vi "Configure Session.vi"(8 "error in":errorcluster, 11 "Plugin in":refnum<class "Sequencer with Output Values.lvclass">) -> (0 "error out":errorcluster, 3 "Plugin out":refnum<class "Sequencer with Output Values.lvclass">)   [LabVIEW 2024, in "Sequencer with Output Values.lvlib" / "Sequencer with Output Values.lvclass"]
uses:
  Sequencer with Output Values.lvclass
  C:/Program Files/National Instruments/LabVIEW 2024/vi.lib/FlexLogger/SDK/PluginSDK.lvlibp/PEFClasses/SDK/Plugin/Plugin.lvclass
  Sequencer with Output Values.lvclass/Sequencer with Output Values.ctl
  Global Strings.vi
  <vilib>/FlexLogger/SDK/PluginSDK.lvlibp/PEFClasses/SDK/Plugin/ParameterAccess/Read I32.vi
  <vilib>/FlexLogger/SDK/PluginSDK.lvlibp/PEFClasses/SDK/Plugin/ParameterAccess/Write I32.vi
  <vilib>/FlexLogger/SDK/PluginSDK.lvlibp/PEFClasses/SDK/Plugin/ParameterAccess/Read DBL.vi
  <vilib>/FlexLogger/SDK/PluginSDK.lvlibp/PEFClasses/SDK/Plugin/ParameterAccess/Read Boolean.vi
  <vilib>/FlexLogger/SDK/PluginSDK.lvlibp/PEFClasses/SDK/Plugin/Plugin.lvclass
  C:/Program Files/National Instruments/LabVIEW 2024/vi.lib/FlexLogger/SDK/PluginSDK.lvlibp/PEFClasses/SDK/Processing Element/Processing Element.lvclass
  C:/dev/niflexlogger-plugins/plugins/Sequencer with Output Values/source/Sequencer with Output Values/Sequencer with Output Values.lvclass
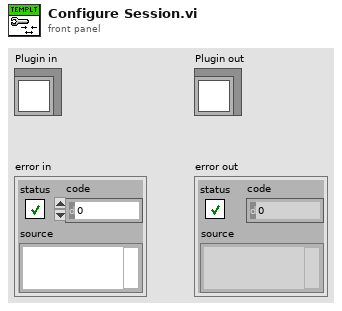
[diagram p1: front panel]
types:
  T1 = typedef "Sequencer with Output Values.lvlib/Sequencer with Output Values.lvclass/Params.ctl" = cluster{"Step Values":T2[], "Only Execute When Test Running":bool, "Current Sequence ID":u32, "Total Iterations":u32, "Last Timestamp":timestamp, "Number of Sequence Steps":i32, "Number of Analog Channels":i32, "Number of Digital Channels":i32, "Delay Before Starting Sequence":dbl}
  T2 = typedef "Step Settings.ctl" = cluster{"Duration":dbl, "Mode":string, "Delay Between Values":dbl, "Analog Values":string[], "Digital Values":string[]}
  T3 = cluster{"Number of Sequence Steps":i32, "Number of Analog Channels":i32, "Number of Digital Channels":i32}
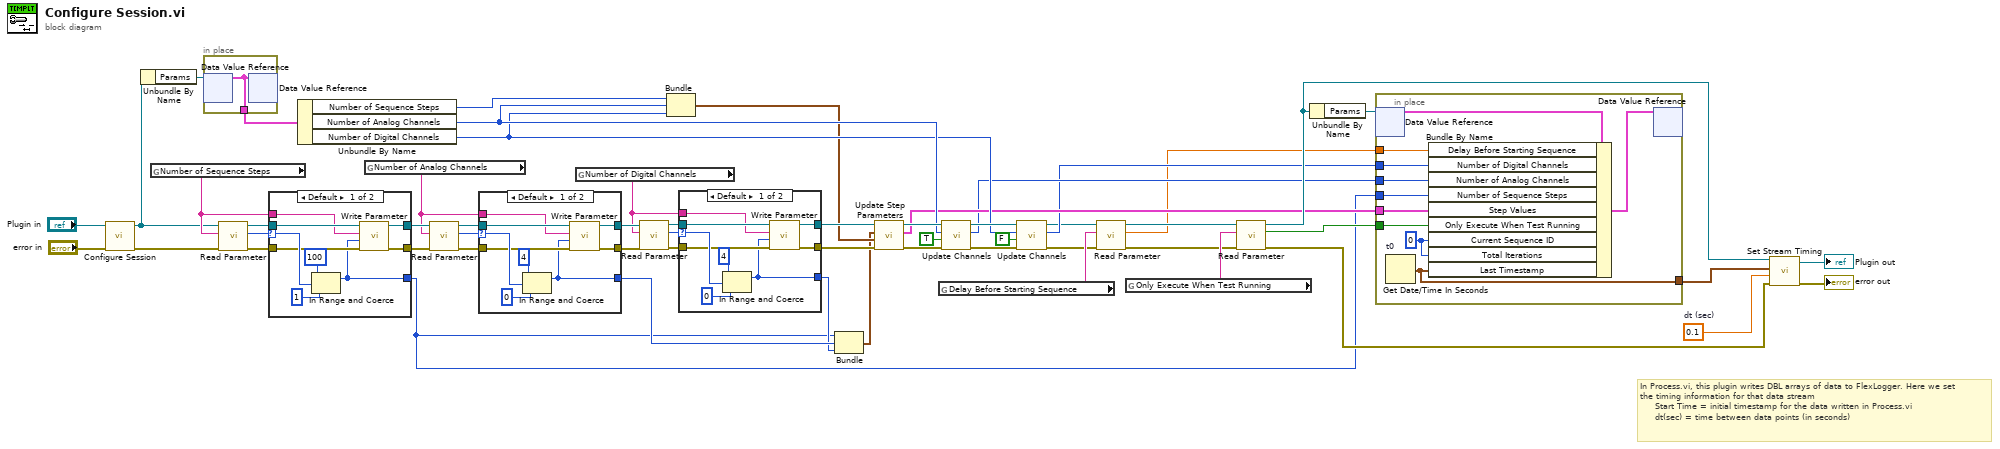
[diagram p0: block diagram]
diagram:
  w50 = 0.1  # dt (sec)
  # "In Process.vi, this plugin writes DBL arrays of data to FlexLogger. Here we set the timing information for that data stream\n     Start Time = initial timestamp for the data written in Process.vi\n     dt(sec) = time between data points (in seconds)"
  n1 = call-parent "Configure Session.vi"("error in (no error)"="error in", "Processing Element in"="Plugin in") -> ("error out"=w12:errorcluster, "Processing Element out"=w13:refnum<class "Sequencer with Output Values.lvclass">)  [unwired: 8 in]
  n2 = Unbundle By Name(w13) -> ("Params"=w46:refnum<data-value>)
  n3 = global read "Global Strings.vi" "Number of Sequence Steps"() -> (w44:string)
  n4 = in-place {
    in-place-border: [w57] -> w11
    n5 = in-place-dvr #1(w46) -> (w57:T1)  [unwired: 1 out]
    n6 = in-place-dvr #1(w57) -> ()  [unwired: 2 out]
  }
  n7 = call-poly <vilib>:"Read Parameter.vi"("error in (no error)"=w12, "Name"=w44, "Plugin in"=w13) -> ("error out"=w43:errorcluster, "Value"=w41:i32, "Plugin out"=w42:refnum<class "Sequencer with Output Values.lvclass">)  [unwired: 5 in, 1 out]
  n8 = case shown="Default" w41 {
    selector: w41 -> [w66 w69]
    tunnel: [w58 w69] -> w7
    tunnel: w42 -> [w63 w68]
    tunnel: [w62 w68] -> w37
    tunnel: w43 -> [w60 w67]
    tunnel: [w61 w67] -> w36
    tunnel: w44 -> [w59 _]
    frame Default {
      n9 = In Range and Coerce(upper limit=100, x=w66, lower limit=1 ("upper limit")) -> (coerced(x)=w58:i32)  [unwired: 1 out]
      n10 = call-poly <vilib>:"Write Parameter.vi"("error in (no error)"=w60, "Value"=w58, "Name"=w59, "Plugin in"=w63) -> ("error out"=w61:errorcluster, "Plugin out"=w62:refnum<class "Sequencer with Output Values.lvclass">)  [unwired: 6 in]
    }
    frame 1..100 {
    }
  }
  n11 = Unbundle By Name(w11) -> ("Number of Sequence Steps"=w18:i32, "Number of Analog Channels"=w17:i32, "Number of Digital Channels"=w16:i32)
  n12 = global read "Global Strings.vi" "Number of Analog Channels"() -> (w29:string)
  n13 = call-poly <vilib>:"Read Parameter.vi"("error in (no error)"=w36, "Name"=w29, "Plugin in"=w37) -> ("error out"=w38:errorcluster, "Value"=w40:i32, "Plugin out"=w39:refnum<class "Sequencer with Output Values.lvclass">)  [unwired: 5 in, 1 out]
  n14 = case shown="Default" w40 {
    selector: w40 -> [w78 w81]
    tunnel: [w70 w81] -> w20
    tunnel: w39 -> [w75 w80]
    tunnel: [w74 w80] -> w32
    tunnel: w38 -> [w72 w79]
    tunnel: [w73 w79] -> w31
    tunnel: w29 -> [w71 _]
    frame Default {
      n15 = In Range and Coerce(upper limit=4, x=w78, lower limit=0 ("upper limit")) -> (coerced(x)=w70:i32)  [unwired: 1 out]
      n16 = call-poly <vilib>:"Write Parameter.vi"("error in (no error)"=w72, "Value"=w70, "Name"=w71, "Plugin in"=w75) -> ("error out"=w73:errorcluster, "Plugin out"=w74:refnum<class "Sequencer with Output Values.lvclass">)  [unwired: 6 in]
    }
    frame 1..100 {
    }
  }
  n17 = global read "Global Strings.vi" "Number of Digital Channels"() -> (w30:string)
  n18 = call-poly <vilib>:"Read Parameter.vi"("error in (no error)"=w31, "Name"=w30, "Plugin in"=w32) -> ("error out"=w35:errorcluster, "Value"=w33:i32, "Plugin out"=w34:refnum<class "Sequencer with Output Values.lvclass">)  [unwired: 5 in, 1 out]
  n19 = Bundle("Number of Sequence Steps"=w18, "Number of Analog Channels"=w17, "Number of Digital Channels"=w16) -> (w15:T3)  [unwired: 1 in]
  n20 = case shown="Default" w33 {
    selector: w33 -> [w90 w93]
    tunnel: [w82 w93] -> w19
    tunnel: w34 -> [w87 w92]
    tunnel: [w86 w92] -> w28
    tunnel: w35 -> [w84 w91]
    tunnel: [w85 w91] -> w27
    tunnel: w30 -> [w83 _]
    frame Default {
      n21 = In Range and Coerce(upper limit=4, x=w90, lower limit=0 ("upper limit")) -> (coerced(x)=w82:i32)  [unwired: 1 out]
      n22 = call-poly <vilib>:"Write Parameter.vi"("error in (no error)"=w84, "Value"=w82, "Name"=w83, "Plugin in"=w87) -> ("error out"=w85:errorcluster, "Plugin out"=w86:refnum<class "Sequencer with Output Values.lvclass">)  [unwired: 6 in]
    }
    frame 1..100 {
    }
  }
  n23 = Bundle("Value"=w7, "Value"=w20, "Value"=w19) -> (w14:cluster{"Value":i32, "Value":i32, "Value":i32})  [unwired: 1 in]
  n24 = call "Update Step Parameters.vi"("error in"=w27, "Old Values"=w15, "New Values"=w14, "Plugin in"=w28) -> ("error out"=w26:errorcluster, "Step Values"=w10:T2[], "Plugin out"=w25:refnum<class "Sequencer with Output Values.lvclass">)  [unwired: 5 in]
  n25 = global read "Global Strings.vi" "Delay Before Starting Sequence"() -> (w6:string)
  n26 = call "Update Channels.vi"("error in"=w26, "Analog"=TRUE, "Previous Number of Channels"=w17, "Plugin in"=w25) -> ("error out"=w22:errorcluster, "Updated Number of Channels"=w9:i32, "Plugin out"=w23:refnum<class "Sequencer with Output Values.lvclass">)  [unwired: 5 in]
  n27 = call "Update Channels.vi"("error in"=w22, "Analog"=FALSE, "Previous Number of Channels"=w16, "Plugin in"=w23) -> ("error out"=w4:errorcluster, "Updated Number of Channels"=w8:i32, "Plugin out"=w5:refnum<class "Sequencer with Output Values.lvclass">)  [unwired: 5 in]
  n28 = call-poly <vilib>:"Read Parameter.vi"("error in (no error)"=w4, "Name"=w6, "Plugin in"=w5) -> ("error out"=w2:errorcluster, "Value"=w1:dbl, "Plugin out"=w3:refnum<class "Sequencer with Output Values.lvclass">)  [unwired: 5 in, 1 out]
  n29 = global read "Global Strings.vi" "Only Execute When Test Running"() -> (w45:string)
  n30 = call-poly <vilib>:"Read Parameter.vi"("error in (no error)"=w2, "Name"=w45, "Plugin in"=w3) -> ("error out"=w51:errorcluster, "Value"=w48:bool, "Plugin out"=w52:refnum<class "Sequencer with Output Values.lvclass">)  [unwired: 5 in, 1 out]
  n31 = Unbundle By Name(w52) -> ("Params"=w49:refnum<data-value>)
  n32 = in-place {
    in-place-border: w48 -> [w101]
    in-place-border: [w99] -> w47
    in-place-border: w10 -> [w98]
    in-place-border: w9 -> [w97]
    in-place-border: w8 -> [w96]
    in-place-border: w7 -> [w95]
    in-place-border: w1 -> [w94]
    w100 = u32 0 ("Current Sequence ID")
    n33 = in-place-dvr #2(w49) -> (w103:T1)  [unwired: 1 out]
    n34 = Get Date/Time In Seconds "t0"() -> (seconds since 1Jan1904=w99:timestamp)
    n35 = Bundle By Name(cluster=w103, "Delay Before Starting Sequence"=w94, "Number of Digital Channels"=w96, "Number of Analog Channels"=w97, "Number of Sequence Steps"=w95, "Step Values"=w98, "Only Execute When Test Running"=w101, "Current Sequence ID"=w100, "Total Iterations"=w100, "Last Timestamp"=w99) -> (w102:T1)
    n36 = in-place-dvr #2(w102) -> ()  [unwired: 2 out]
  }
  n37 = call-dynamic "Set Stream Timing.vi"("error in (no error)"=w51, "dt(sec)"=w50, "Start Time"=w47, "Plugin in"=w52) -> ("error out"=→"error out":errorcluster, "Plugin out"=→"Plugin out":refnum<class "Sequencer with Output Values.lvclass">)  [unwired: 6 in]
